vi "resample.vi"(11 "Array in":u8[](array[numeric])) -> (3 "Array out":u32[](array[numeric]))   [LabVIEW 2018]
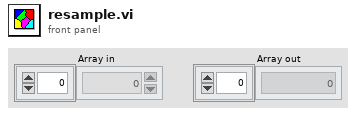
[diagram p1: front panel]
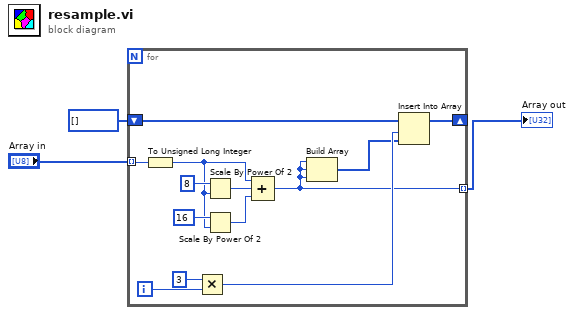
[diagram p0: block diagram]
diagram:
  n1 = for {
    tunnel: "Array in" -> [w11] mode=indexing
    shift-right: [w16] -> _
    shift-left: u32[] [] ("Array in") -> [w12]
    tunnel: [w4] -> w1 mode=indexing
    i -> [w15]
    n2 = To Unsigned Long Integer(number=w11) -> (unsigned 32bit integer=w6:u32)
    n3 = Multiply(x=3, y=w15) -> (x*y=w13:i32)
    n4 = Scale By Power Of 2(n=i16 8, x=w6) -> (x*2^n=w7:u32)
    n5 = Scale By Power Of 2(n=i16 16, x=w6) -> (x*2^n=w8:u32)
    n6 = Compound Arithmetic op=ADD(w6, w7, w8) -> (w4:u32)
    n7 = Build Array(w4, w4, w4) -> (w5:u32[])
    n8 = Insert Into Array(array=w12, index=w13, new element=w5) -> (w16:u32[])
  }
  "Array out" <- w1
